vi "isAnalysisRunning.vi"(8 "error in (no error)":errorcluster, 11 "ImageStreamViewer in":refnum<class "ImageStreamViewer.lvclass">) -> (0 "error out":errorcluster, 2 "running?":bool, 3 "ImageStreamViewer out":refnum<class "ImageStreamViewer.lvclass">)   [LabVIEW 2009, in "Views.lvlib" / "Camera.lvlib" / "ImageStreamViewer.lvclass"]
uses:
  ImageStreamViewer.lvclass
  ImageStreamViewer.lvclass/ImageStreamViewer.ctl
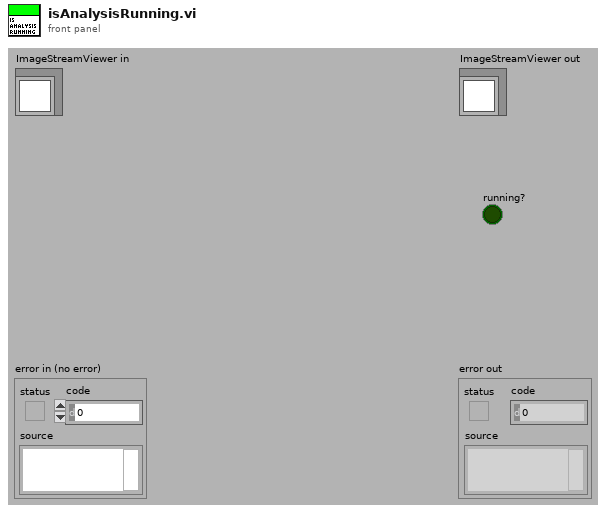
[diagram p1: front panel]
types:
  T1 = enum32{"Bad", "Idle", "Run top level", "Running"}
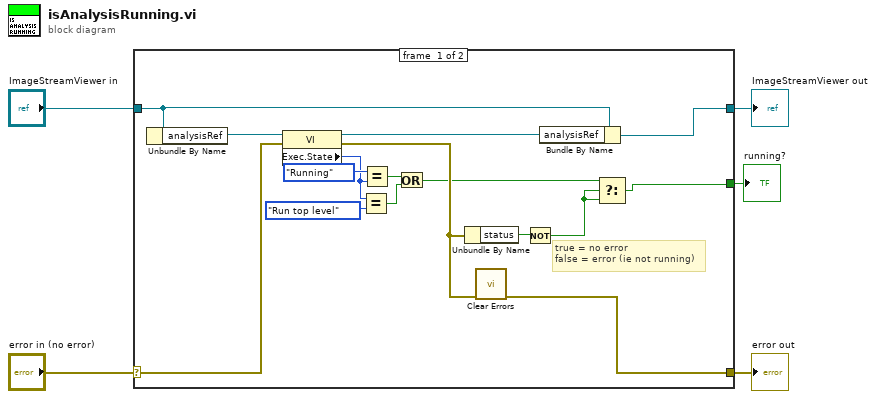
[diagram p0: block diagram]
diagram:
  n1 = case shown="No Error" "error in (no error)" {
    selector: "error in (no error)" -> [w18 w23]
    tunnel: [w19 w23] -> w4
    tunnel: [w15 w22] -> w2
    tunnel: "ImageStreamViewer in" -> [w16 w22]
    tunnel: [w6 _] -> w1
    frame #0 {
      # "true = no error\nfalse = error (ie not running)"
      n2 = Unbundle By Name(w16) -> ("analysisRef"=w21:refnum<vi>)
      n3 = property class="VI"(reference=w21, error in=w18) -> (reference out=w14:refnum<vi>, error out=w20:errorcluster, "Exec.State"=w12:T1)
      n4 = Equal?(x=w12, y=T1."Run top level" ("Execution:State")) -> (x = y?=w9:bool)
      n5 = Equal?(x=T1."Running" ("Execution:State"), y=w12) -> (x = y?=w10:bool)
      n6 = Or(x=w10, y=w9) -> (x .or. y?=w8:bool)
      n7 = Unbundle By Name(w20) -> ("status"=w17:bool)
      n8 = call <vilib>:"Clear Errors.vi"("error in (no error)"=w20) -> ("error out"=w19:errorcluster)  [unwired: 6 in]
      n9 = Not(x=w17) -> (.not. x?=w7:bool)
      n10 = Bundle By Name(cluster=w16, "analysisRef"=w14) -> (w15:refnum<class "ImageStreamViewer.lvclass">)
      n11 = Select(t=w8, s=w7, f=w7) -> (s? t:f=w6:bool)
    }
    frame #1 {
    }
  }
  "error out" <- w4
  "ImageStreamViewer out" <- w2
  "running?" <- w1
